vi "ASI Get ID.vi"(10 "pID":T1, 11 "iCameraID":i32) -> (2 "pID out":T1, 3 "function return":i32)   [LabVIEW 2023, in "ASICamera2_no_err.lvlib"]
doc: "ASICAMERA_API ASI_ERROR_CODE ASIGetID(int iCameraID, ASI_ID* pID);"
uses:
  ASICamera2_no_err.lvlib
  ASICamera2.dll
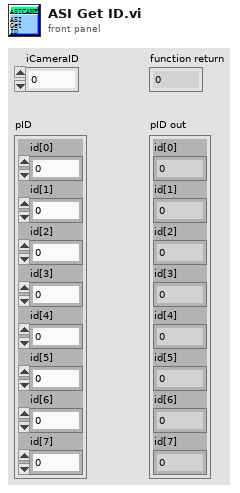
[diagram p1: front panel]
types:
  T1 = cluster{"id[0]":u8, "id[1]":u8, "id[2]":u8, "id[3]":u8, "id[4]":u8, "id[5]":u8, "id[6]":u8, "id[7]":u8}
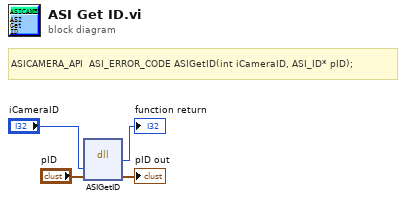
[diagram p0: block diagram]
diagram:
  # "ASICAMERA_API  ASI_ERROR_CODE ASIGetID(int iCameraID, ASI_ID* pID);"
  n1 = dll-call lib="C:/Users/quantum/Documents/LVDAQ/ConcreteClasses/ConcreteInstrumentClasses/CameraClasses/ZWO_ASI_LV/Labview_ASI_demo_64bit_221128/user.lib/ASICamera2_no_err/ASICamera2.*" fn="ASIGetID"("iCameraID"="iCameraID", "pID"="pID") -> (→"function return":i32, "pID"=→"pID out":T1)  [unwired: 4 in, 2 out]
